vi "ExtractTreeCluster.vi"(8 "error in (no error)":errorcluster, 10 "NumberOfColumns":i32=4, 11 "TreeReference":refnum<vi>) -> (0 "error out":errorcluster, 1 "All Tags":string[](array[string]), 2 "TreeCluster":T1(array[cluster]), 3 "TreeReference":refnum<vi>)   [LabVIEW 2013, in "FindName Task_Manager.lvlib"]
uses:
  FindName Task_Manager.lvlib
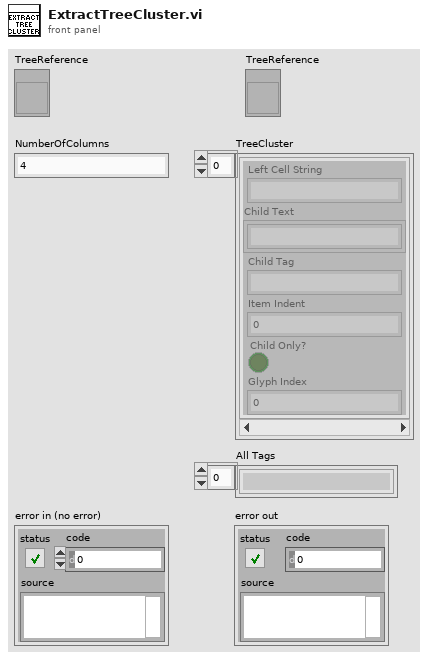
[diagram p1: front panel]
types:
  T1 = cluster{"Left Cell String":string, "Child Text":string[], "Child Tag":string, "Item Indent":i32, "Child Only?":bool, "Glyph Index":i32}[]
  T2 = cluster{"Left Cell String":string, "Child Text":string[], "Child Tag":string, "Item Indent":i32, "Child Only?":bool, "Glyph Index":i32}
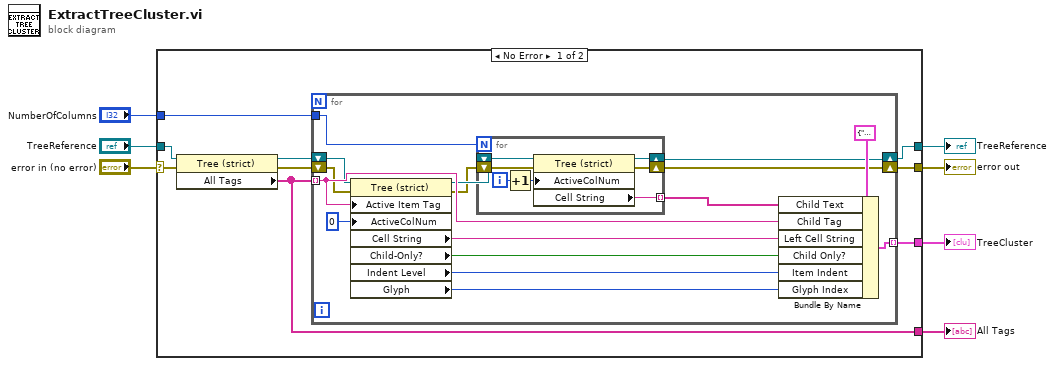
[diagram p0: block diagram]
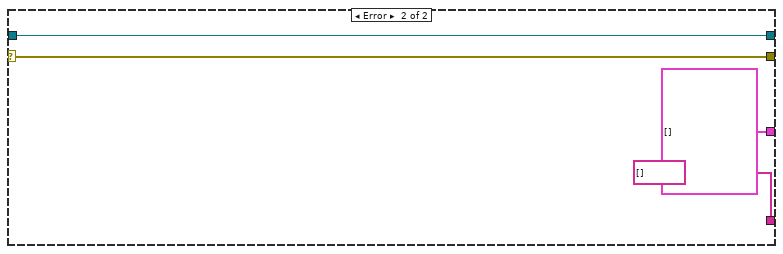
[diagram p2: hidden frame]
diagram:
  n1 = case shown="No Error" "error in (no error)" {
    selector: "error in (no error)" -> [w11 w43]
    tunnel: [w16 T1 []] -> w7
    tunnel: "NumberOfColumns" -> [w15 _]
    tunnel: "TreeReference" -> [w14 w42]
    tunnel: [w12 w42] -> w4
    tunnel: [w9 w43] -> w2
    tunnel: [w8 string[] [] ("All Tags")] -> w1
    frame No Error {
      n2 = property on="Property Node" class="Tree (strict)"(reference=w14, error in=w11) -> (reference out=w13:refnum<vi>, error out=w10:errorcluster, "All Tags"=w8:string[])
      n3 = for {
        tunnel: w8 -> [w27] mode=indexing
        tunnel: [w31] -> w16 mode=indexing
        tunnel: w15 -> [w28]
        shift-right: [w21] -> w12
        shift-left: w13 -> [w18]
        shift-right: [w20] -> w9
        shift-left: w10 -> [w17]
        n4 = property on="Property Node" class="Tree (strict)"(reference=w18, error in=w17, "Active Item Tag"=w27, "ActiveColNum"=0 ("Active Cell:Active Column Number")) -> (reference out=w23:refnum<vi>, error out=w22:errorcluster, "Cell String"=w30:string, "Child-Only?"=w25:bool, "Indent Level"=w26:i32, "Glyph"=w32:i32)
        n5 = for {
          N: w28 -> [_]
          tunnel: [w37] -> w19 mode=indexing
          shift-right: [w35] -> w21
          shift-left: w23 -> [w36]
          shift-right: [w33] -> w20
          shift-left: w22 -> [w34]
          i -> [w39]
          n6 = Increment(x=w39) -> (x+1=w38:i32)
          n7 = property on="Property Node" class="Tree (strict)"(reference=w36, error in=w34, "ActiveColNum"=w38) -> (reference out=w35:refnum<vi>, error out=w33:errorcluster, "Cell String"=w37:string)
        }
        n8 = Bundle By Name(cluster=T2 {"Left Cell String"="", "Child Text"=[], "Child Tag"="", "Item Indent"=0, "Child Only?"=FALSE, "Glyph Index"=0} ("Item"), "Child Text"=w19, "Child Tag"=w27, "Left Cell String"=w30, "Child Only?"=w25, "Item Indent"=w26, "Glyph Index"=w32) -> (w31:T2)
      }
    }
    frame Error {
    }
  }
  "TreeCluster" <- w7
  "TreeReference" <- w4
  "error out" <- w2
  "All Tags" <- w1
